vi "NI OCR-Import Picture.vi"(8 "error in":errorcluster, 11 "Buffer Data In":T1={"VI Refnum"=refnum, "Src Image"=refnum, "Dst Image"=refnum, "Ctl Refnum []"=[], "Ctl Label"=[], "User Event"=refnum, "Event Registration Refnum"=refnum, "Timeout"=0, "IMAQ OCR Session"=refnum, "Objects"=[], "ROI Descriptor"={"Global Rectangle"=[], "Contours"=[]}, "Settings"={"Objects"=0, "Threshold"=128, "Reject Border"=FALSE, "Fill Holes"=FALSE, "Min Object Size"=FALSE, "Min Size"=3, "Max Object Size"=FALSE, "Max Size"=100, "Show Search Area"=FALSE, "Show Center"=TRUE, "Show Bounding Box"=TRUE}} {"Settings"."Objects" items=["Bright Objects", "Dark Objects"]; "Settings"."Threshold" min=1 max=999999999 step=1; "Settings"."Max Size" min=1 max=999999999 step=1; "Settings"."Min Size" min=1 max=999999999 step=1; "ROI Descriptor"."Contours"."Type" items=["No Selection", "Point", "Line", "Rectangle", "Oval", "Polygon", "Freehand Region", "Annulus", "Unused2", "Unused3", "Broken Line", "Freehand Line", "Rotated Rectangle"]; "Objects"."Aspect Ratio" format="%.2f"; "Objects"."Orientation" format="%.2f"; "Objects"."Area" format="%.2f"; "Objects"."Object Center"."Y" format="%.2f"; "Objects"."Object Center"."X" format="%.2f"}) -> (0 "error out":errorcluster, 3 "Buffer Data Out":T1={"VI Refnum"=refnum, "Src Image"=refnum, "Dst Image"=refnum, "Ctl Refnum []"=[], "Ctl Label"=[], "User Event"=refnum, "Event Registration Refnum"=refnum, "Timeout"=0, "IMAQ OCR Session"=refnum, "Objects"=[], "ROI Descriptor"={"Global Rectangle"=[], "Contours"=[]}, "Settings"={"Objects"=0, "Threshold"=128, "Reject Border"=FALSE, "Fill Holes"=FALSE, "Min Object Size"=FALSE, "Min Size"=3, "Max Object Size"=FALSE, "Max Size"=100, "Show Search Area"=FALSE, "Show Center"=TRUE, "Show Bounding Box"=TRUE}} {"Settings"."Objects" items=["Bright Objects", "Dark Objects"]; "Settings"."Threshold" min=1 max=999999999 step=1; "Settings"."Max Size" min=1 max=999999999 step=1; "Settings"."Min Size" min=1 max=999999999 step=1; "ROI Descriptor"."Contours"."Type" items=["No Selection", "Point", "Line", "Rectangle", "Oval", "Polygon", "Freehand Region", "Annulus", "Unused2", "Unused3", "Broken Line", "Freehand Line", "Rotated Rectangle"]; "Objects"."Aspect Ratio" format="%.2f"; "Objects"."Orientation" format="%.2f"; "Objects"."Area" format="%.2f"; "Objects"."Object Center"."Y" format="%.2f"; "Objects"."Object Center"."X" format="%.2f"})   [LabVIEW 2016]
uses:
  Data Def/NI OCR-Buffer Data.ctl
  <vilib>/vision/Image Controls.llb/IMAQ Image.ctl
  Data Def/NI OCR-User Event Data.ctl
  <vilib>/vision/OCR.llb/IMAQ OCR Session.ctl
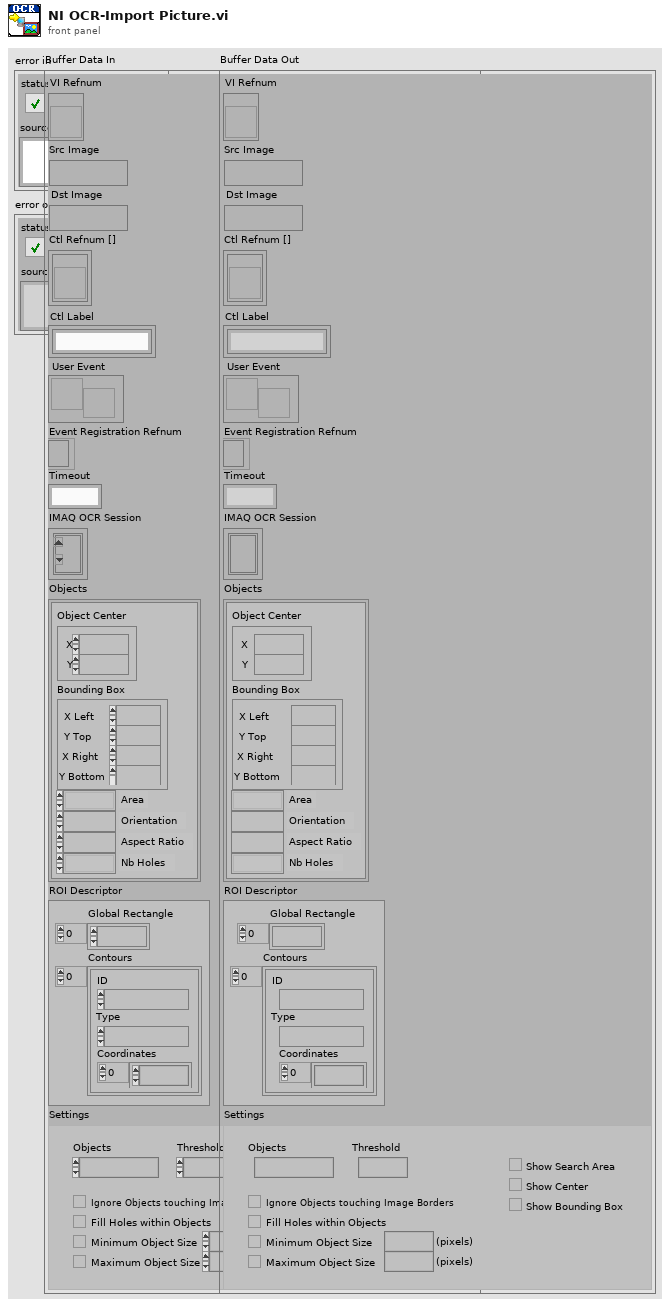
[diagram p1: front panel]
types:
  T1 = typedef "NI OCR-Buffer Data.ctl" = cluster{"VI Refnum":refnum<vi>, "Src Image":T2, "Dst Image":T2, "Ctl Refnum []":refnum<vi>[], "Ctl Label":string[], "User Event":refnum<user-event>, "Event Registration Refnum":refnum<event-registration>, "Timeout":i32, "IMAQ OCR Session":T3, "Objects":cluster{"Object Center":cluster{"X":sgl, "Y":sgl}, "Bounding Box":cluster{"X Left":i32, "Y Top":i32, "X Right":i32, "Y Bottom":i32}, "Area":sgl, "Orientation":sgl, "Aspect Ratio":sgl, "Nb Holes":i32}[], "ROI Descriptor":T4, "Settings":cluster{"Objects":u16, "Threshold":i32, "Reject Border":bool, "Fill Holes":bool, "Min Object Size":bool, "Min Size":i32, "Max Object Size":bool, "Max Size":i32, "Show Search Area":bool, "Show Center":bool, "Show Bounding Box":bool}}
  T2 = typedef "IMAQ Image.ctl" = refnum<image>
  T3 = typedef "IMAQ OCR Session.ctl" = refnum<k1>
  T4 = typedef "ROI Descriptor" = cluster{"Global Rectangle":i32[], "Contours":cluster{"ID":enum32{"External", "Internal"}, "Type":u32, "Coordinates":i32[]}[]}
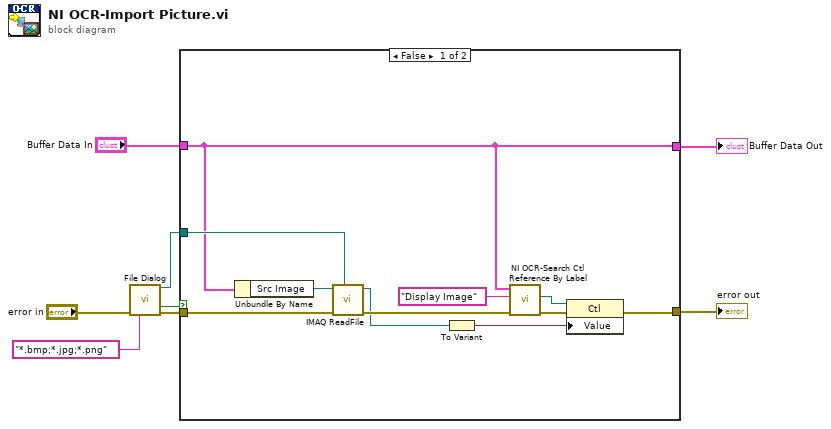
[diagram p0: block diagram]
diagram:
  n1 = call "File Dialog"("error in"="error in", "pattern (all files)"="*.bmp;*.jpg;*.png") -> ("selected path"=w4:path, "cancelled"=w5:bool, "error out"=w6:errorcluster)  [unwired: 10 in, 1 out]
  n2 = case shown="False" w5 {
    tunnel: w6 -> [w19 _]
    tunnel: w4 -> [w18 _]
    tunnel: "Buffer Data In" -> [w9 w20]
    tunnel: [w10 _] -> w2
    tunnel: [w9 w20] -> w1
    frame False {
      n3 = Unbundle By Name(w9) -> ("Src Image"=w17:T2)
      n4 = call "IMAQ ReadFile"("File Path"=w18, "error in (no error)"=w19, "Image"=w17) -> ("error out"=w16:errorcluster, "Image Out"=w12:T2)  [unwired: 4 in, 3 out]
      n5 = To Variant(anything=w12) -> (Variant=w11:variant)
      n6 = call "NI OCR-Search Ctl Reference By Label.vi"("error in"=w16, "Ctl Label"="Display Image", "Buffer Data In"=w9) -> ("error out"=w14:errorcluster, "Ctl Refnum"=w13:refnum<vi>)  [unwired: 5 in, 2 out]
      n7 = property class="Ctl"(reference=w13, error in=w14, "Value"=w11) -> (error out=w10:errorcluster)  [unwired: 1 out]
    }
    frame True {
    }
  }
  "error out" <- w2
  "Buffer Data Out" <- w1
